vi "Read Coils Response.vi"(8 "error in (no error)":errorcluster, 10 "Modbus data unit in":refnum<class "Modbus Data Unit (PDU).lvclass">) -> (0 "error out":errorcluster, 2 "data":bool[](array[boolean]))   [LabVIEW 2017, in "SubVIs.lvlib" / "Master Function Definition.lvlib"]
doc: "Decodes the response for the read coils function."
uses:
  <vilib>/Modbus/subvis/Data and Functions/Master Function Definition/Master Function Definition.lvlib
  <vilib>/Modbus/subvis/Modbus Data Unit (PDU)/Modbus Data Unit (PDU).lvclass
  <vilib>/Modbus/subvis/SubVIs.lvlib
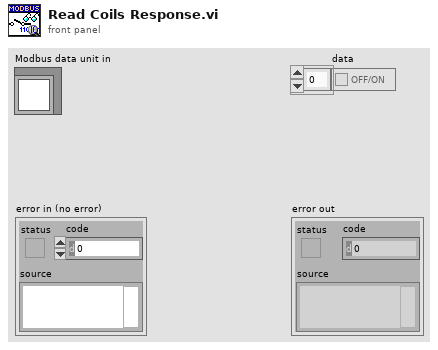
[diagram p1: front panel]
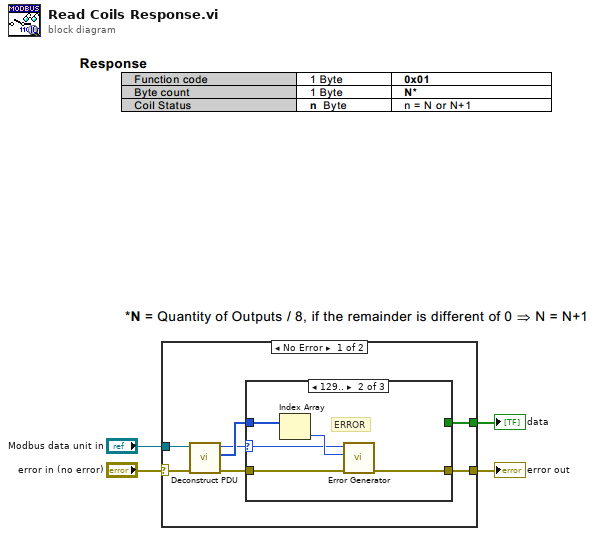
[diagram p0: block diagram]
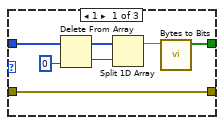
[diagram p2: hidden frame]
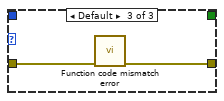
[diagram p3: hidden frame]
diagram:
  n1 = case shown="No Error" "error in (no error)" {
    selector: "error in (no error)" -> [w5 w26]
    tunnel: [w11 w26] -> w4
    tunnel: "Modbus data unit in" -> [w8 _]
    tunnel: [w10 _] -> w2
    frame No Error {
      n2 = call <vilib>:"Deconstruct PDU.vi"("error in (no error)"=w5, "Modbus data unit in"=w8) -> ("error out"=w7:errorcluster, "data"=w9:u8[], "function"=w6:u8)  [unwired: 7 in]
      n3 = case shown="129.." w6 {
        selector: w6 -> [_ w19 _]
        tunnel: w7 -> [w16 w20 w25]
        tunnel: w9 -> [w18 w23 _]
        tunnel: [w16 w22 w24] -> w11
        tunnel: [w17 _ _] -> w10
        frame 1 {
          n4 = Delete From Array(array=w18, index=0) -> (deleted portion=w14:u8, array with subset deleted=w13:u8[])  [unwired: 1 in]
          n5 = Split 1D Array(array=w13, index=w14) -> (first subarray=w15:u8[])  [unwired: 1 out]
          n6 = call <vilib>:"Bytes to Bits.vi"("bytes"=w15) -> ("bits"=w17:bool[])  [unwired: 10 in]
        }
        frame 129.. {
          # "ERROR"
          n7 = Index Array(array=w23) -> (element=w21:u8)  [unwired: 1 in]
          n8 = call <vilib>:"Error Generator.vi"("error in (no error)"=w20, "data return (error code)"=w21, "function return"=w19) -> ("error out"=w22:errorcluster)  [unwired: 8 in]
        }
        frame Default {
          n9 = call <vilib>:"Function code mismatch error.vi"("error in (no error)"=w25) -> ("error out"=w24:errorcluster)  [unwired: 10 in]
        }
      }
    }
    frame Error {
    }
  }
  "error out" <- w4
  "data" <- w2
